vi "CopyMap.vi"(8 "error in (no error)":errorcluster, 9 "data flow":T1, 10 "data event config":T5) -> (0 "error out":errorcluster, 2 "data event config out":T5)   [LabVIEW 2017, in "EmsaDataEventCreator.lvlib"]
uses:
  <vilib>/addons/InsightCM/Devices/Shared/Emsa/EmsaDataEventCreator/EmsaDataEventCreator.lvlib
  <vilib>/addons/InsightCM/Devices/Shared/Emsa/EmsaDataEventCreator/controls/DataEventConfig.ctl
  <vilib>/addons/PointValueMap/controls/PointMap.ctl
  <vilib>/addons/InsightCM/Devices/Shared/Emsa/EmsaDataEventCreator/controls/SweepParams.ctl
  <vilib>/addons/InsightCM/Devices/Shared/Common/DataFlow/controls/Data.ctl
  <vilib>/addons/InsightCM/Utilities/DataAccessors/controls/wfmSGL_DVR.ctl
  <vilib>/addons/InsightCM/Devices/Shared/Common/DataFlow/controls/Type.ctl
  <vilib>/addons/PointValueMap/PointValueMap.lvlib
  <vilib>/addons/InsightCM/Devices/Shared/Common/DataFlow/DataFlow.lvlib
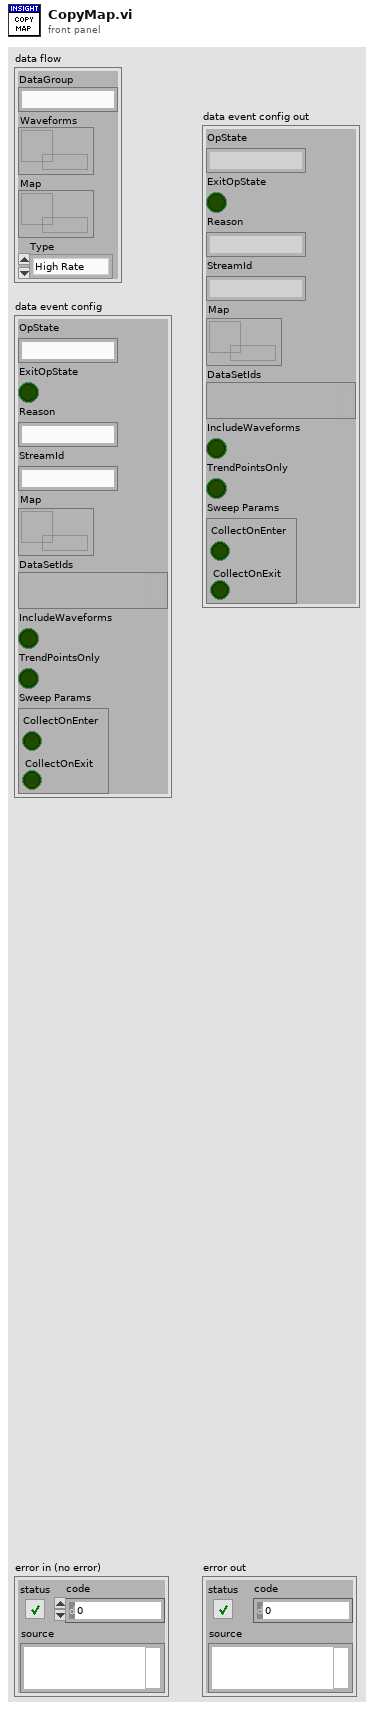
[diagram p1: front panel]
types:
  T1 = typedef "DataFlow.lvlib/Data.ctl" = cluster{"DataGroup":string, "Waveforms":T2, "Map":T3, "Type":T4}
  T2 = typedef "wfmSGL_DVR.ctl" = refnum<data-value>
  T3 = typedef "PointValueMap.lvlib/PointMap.ctl" = refnum<data-value>
  T4 = typedef "DataFlow.lvlib/Type.ctl" = enum16{"High Rate", "Low Rate", "Burst Mode"}
  T5 = typedef "EmsaDataEventCreator.lvlib/DataEventConfig.ctl" = cluster{"OpState":string, "ExitOpState":bool, "Reason":string, "StreamId":string, "Map":T3, "DataSetIds":variant, "IncludeWaveforms":bool, "TrendPointsOnly":bool, "Sweep Params":T6}
  T6 = typedef "EmsaDataEventCreator.lvlib/SweepParams.ctl" = cluster{"CollectOnEnter":bool, "CollectOnExit":bool}
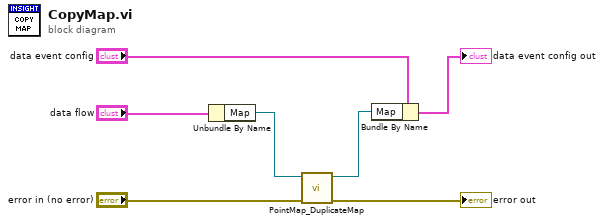
[diagram p0: block diagram]
diagram:
  n1 = Unbundle By Name("data flow") -> ("Map"=w3:T3)
  n2 = call <vilib>:"PointMap_DuplicateMap.vi"("error in (no error)"="error in (no error)", "map in"=w3) -> ("error out"=→"error out":errorcluster, "duplicate map"=w6:T3)  [unwired: 8 in]
  n3 = Bundle By Name(cluster="data event config", "Map"=w6) -> (→"data event config out":T5)
